vi "Get NI-DAQ Data.vi"(8 "error in (no error)":errorcluster, 10 "samples per channel":i32=220000, 11 "task":refnum<k21>) -> (0 "error out":errorcluster, 2 "data":waveform(dbl)[](array[waveform]), 3 "task out":refnum<k21>)   [LabVIEW 2015]
uses:
  <vilib>/DAQmx/read.llb/DAQmx Read (Analog 1D Wfm NChan NSamp).vi
  <vilib>/DAQmx/miscellaneous.llb/DAQmx Fill In Error Info.vi
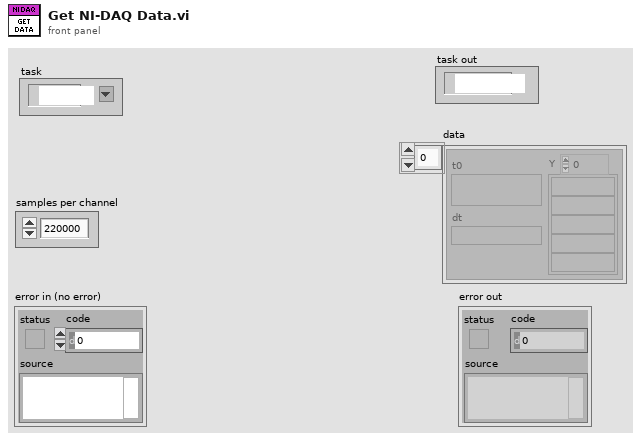
[diagram p1: front panel]
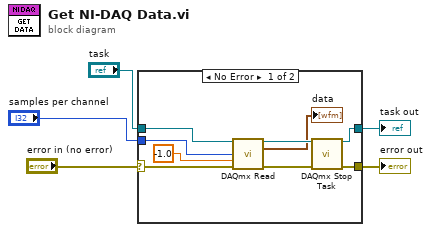
[diagram p0: block diagram]
diagram:
  n1 = case shown="No Error" "error in (no error)" {
    selector: "error in (no error)" -> [w13 w16]
    tunnel: [w9 w16] -> w4
    tunnel: [w7 w15] -> w3
    tunnel: "task" -> [w8 w15]
    tunnel: "samples per channel" -> [w6 _]
    frame No Error {
      n2 = call-poly <vilib>:"DAQmx Read.vi"("task/channels in"=w8, "number of samples per channel"=w6, "timeout"=-1.0, "error in"=w13) -> ("task out"=w12:refnum<k21>, "data"=→"data":waveform(dbl)[], "error out"=w10:errorcluster)  [unwired: 9 in]
      n3 = call <vilib>:"DAQmx Stop Task.vi"("task/channels in"=w12, "error in"=w10) -> ("task out"=w7:refnum<k21>, "error out"=w9:errorcluster)  [unwired: 12 in]
    }
    frame Error {
    }
  }
  "error out" <- w4
  "task out" <- w3
